vi "Get Encoder Value From User.vi"(8 "error in (no error)":errorcluster, 11 "Encoder in":refnum<class "Encoder.lvclass">) -> (0 "error out":errorcluster, 3 "Numeric":i32)   [LabVIEW 2014]
uses:
  <vilib>/LabVIEW Universal Transcriptor/LabVIEW Universal Transcriptor Rotary Encoder Library/Encoder.lvclass
  <vilib>/LabVIEW Universal Transcriptor/LabVIEW to Arduino Transcriptor/Transcriptors/System API/Serial println string.vi
  <vilib>/LabVIEW Universal Transcriptor/LabVIEW for Arduino Math Library/Arduino Math.lvlib
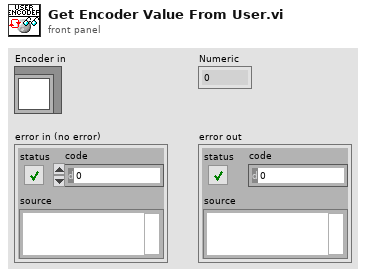
[diagram p1: front panel]
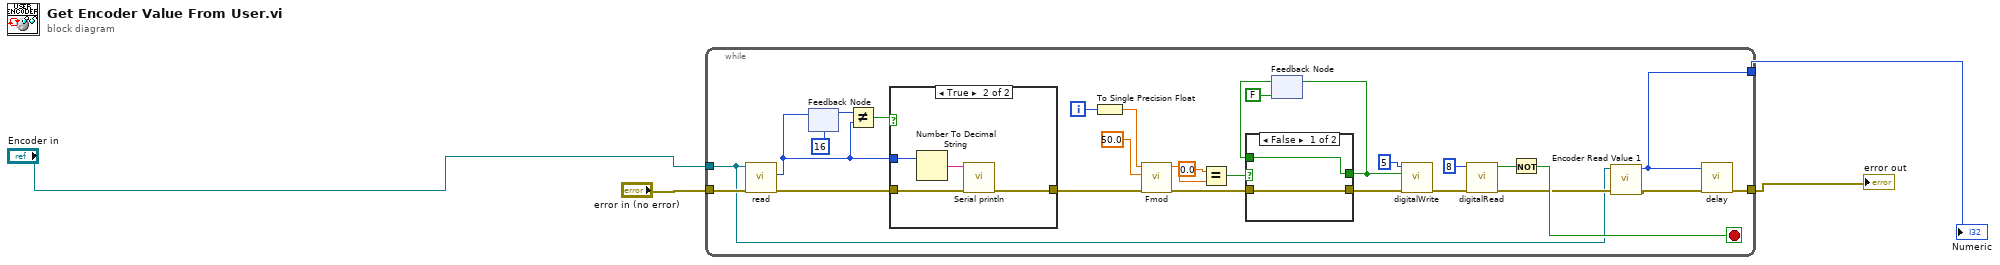
[diagram p0: block diagram]
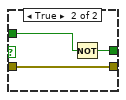
[diagram p3: hidden frame]
diagram:
  n1 = while {
    tunnel: [w13] -> w3
    tunnel: "Encoder in" -> [w5]
    tunnel: "error in (no error)" -> [w32]
    tunnel: [w6] -> w2
    i -> [w28]
    stop <- w10 stop-if-true
    n2 = call <vilib>:"read.vi"("error in (no error)"=w32, "Encoder in"=w5) -> ("error out"=w16:errorcluster, "value"=w9:i32)  [unwired: 7 in]
    n3 = feedback-in #1(w9) -> ()
    n4 = feedback #1(16 ("value")) -> (w15:i32)
    n5 = Not Equal?(x=w15, y=w9) -> (x != y?=w14:bool)
    n6 = case shown="True" w14 {
      tunnel: [w33 w36] -> w27
      tunnel: w16 -> [w33 w35]
      tunnel: w9 -> [_ w34]
      frame False {
      }
      frame True {
        n7 = Number To Decimal String(number=w34) -> (decimal integer string=w37:string)  [unwired: 1 in]
        n8 = call-poly <vilib>:"Serial println.vi"("Error In"=w35, "string in"=w37) -> ("Error Out"=w36:errorcluster)  [unwired: 9 in]
      }
    }
    n9 = To Single Precision Float(number=w28) -> (single precision float=w29:sgl)
    n10 = call <vilib>:"Fmod.vi"("Error In"=w27, "y"=sgl 50.0, "x"=w29) -> ("Error Out"=w26:errorcluster, "fmod(x,y)"=w23:sgl)  [unwired: 7 in]
    n11 = Equal?(x=sgl 0.0, y=w23) -> (x = y?=w24:bool)
    n12 = feedback #2(FALSE) -> (w22:bool)
    n13 = case shown="False" w24 {
      tunnel: w26 -> [w38 w40]
      tunnel: [w39 w42] -> w17
      tunnel: w22 -> [w39 w41]
      tunnel: [w38 w40] -> w18
      frame False {
      }
      frame True {
        n14 = Not(x=w41) -> (.not. x?=w42:bool)
      }
    }
    n15 = feedback-in #2(w17) -> ()
    n16 = call <vilib>:"digitalWrite.vi"("Error In"=w18, "value"=w17, "pin number"=5) -> ("Error Out"=w19:errorcluster)  [unwired: 8 in]
    n17 = call <vilib>:"digitalRead.vi"("Error In"=w19, "pin number"=8) -> ("Error Out"=w8:errorcluster, "value"=w11:bool)  [unwired: 8 in]
    n18 = Not(x=w11) -> (.not. x?=w10:bool)
    n19 = call "Encoder Read Value 1.vi"("error in (no error)"=w8, "Encoder in"=w5) -> ("error out"=w7:errorcluster, "Numeric"=w6:i32)  [unwired: 8 in]
    n20 = call <vilib>:"delay.vi"("Error In"=w7, "time (ms)"=w6) -> ("Error Out"=w13:errorcluster)  [unwired: 9 in]
  }
  "error out" <- w3
  "Numeric" <- w2
